vi "UserManage.vi"() -> ()   [LabVIEW 2011]
uses:
  Global/Globalclient.vi
panel:
  out "删除用户":string
  out "已登陆":string[][](table)
  in  "stop":bool
  out "未登陆":string[][](table)
  out "连接数":u8
  in  "Add Button":bool
  in  "Remove Button":bool
  out "射频":string[][](table)
  out "时钟":string[][](table)
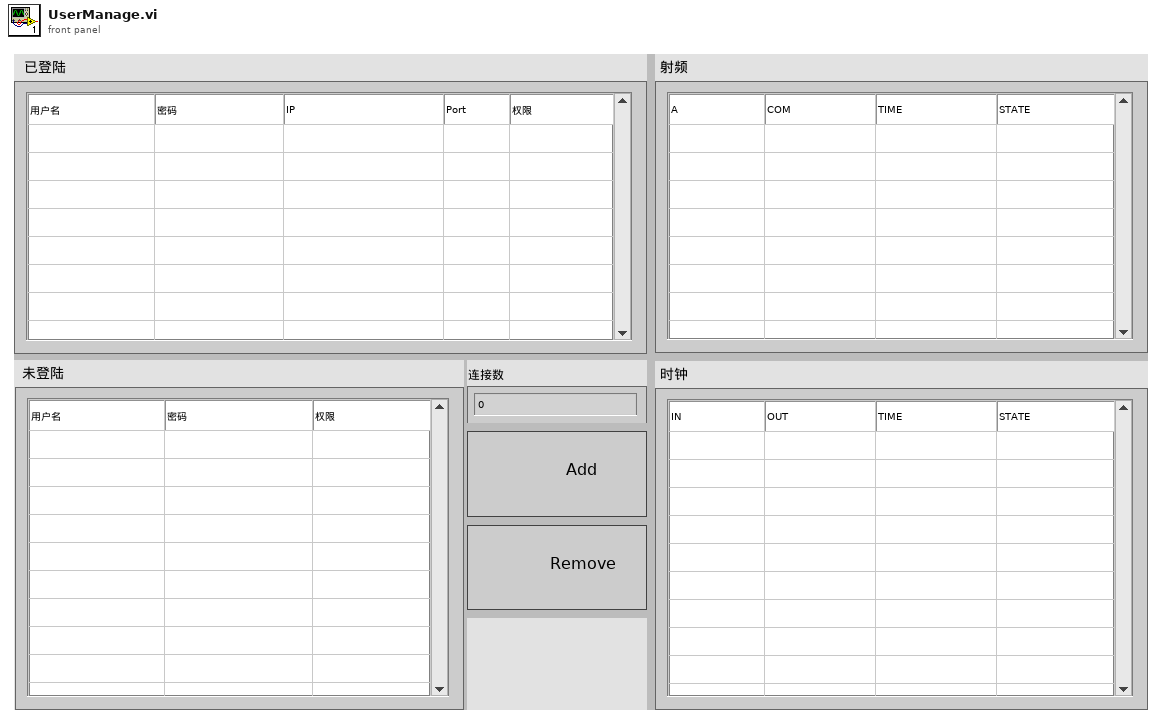
[diagram p1: front panel]
types:
  T1 = enum16{"Standard", "Buffered", "CRLF", "Immediate"}
  T2 = typedef "LVPoint32TypeDef.ctl" = cluster{"Horizontal":i32, "Vertical":i32}
  T3 = typedef "LVRowAndColumnTypeDef.ctl" = cluster{"Row":i32, "Column":i32}
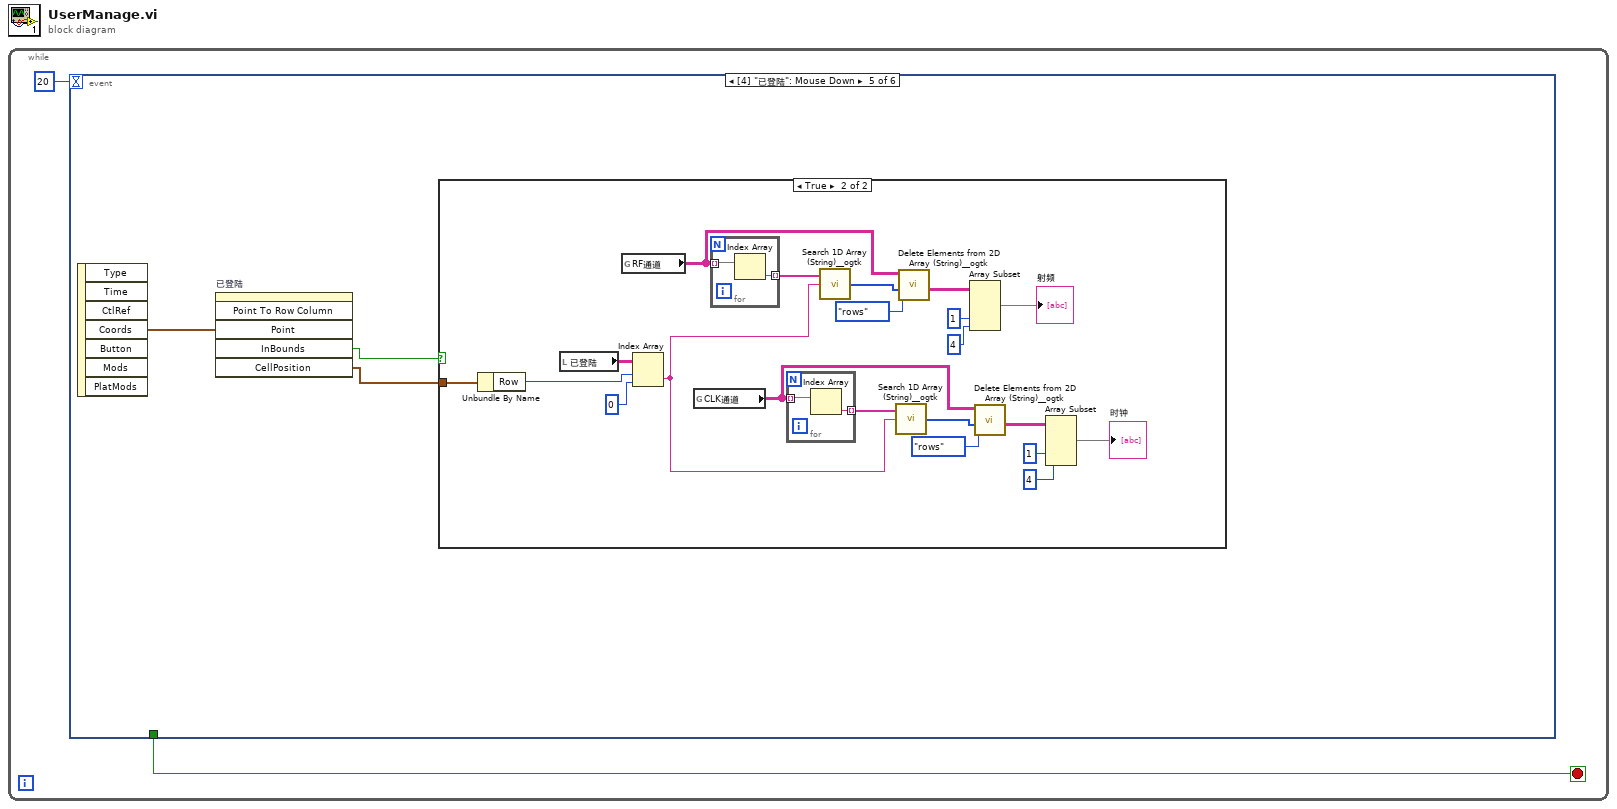
[diagram p0: block diagram]
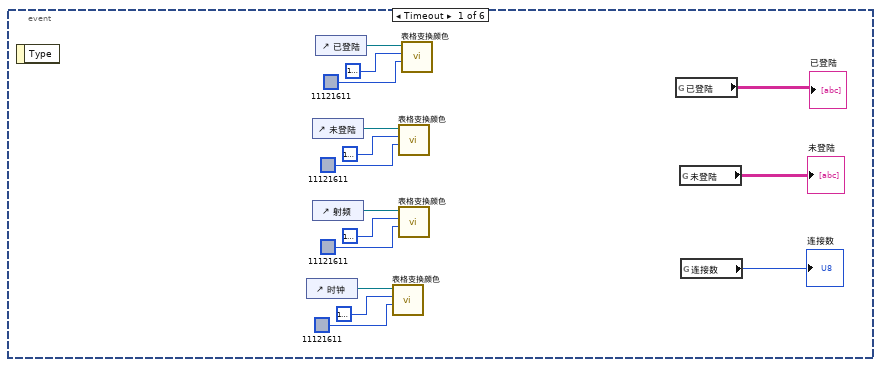
[diagram p2: hidden frame]
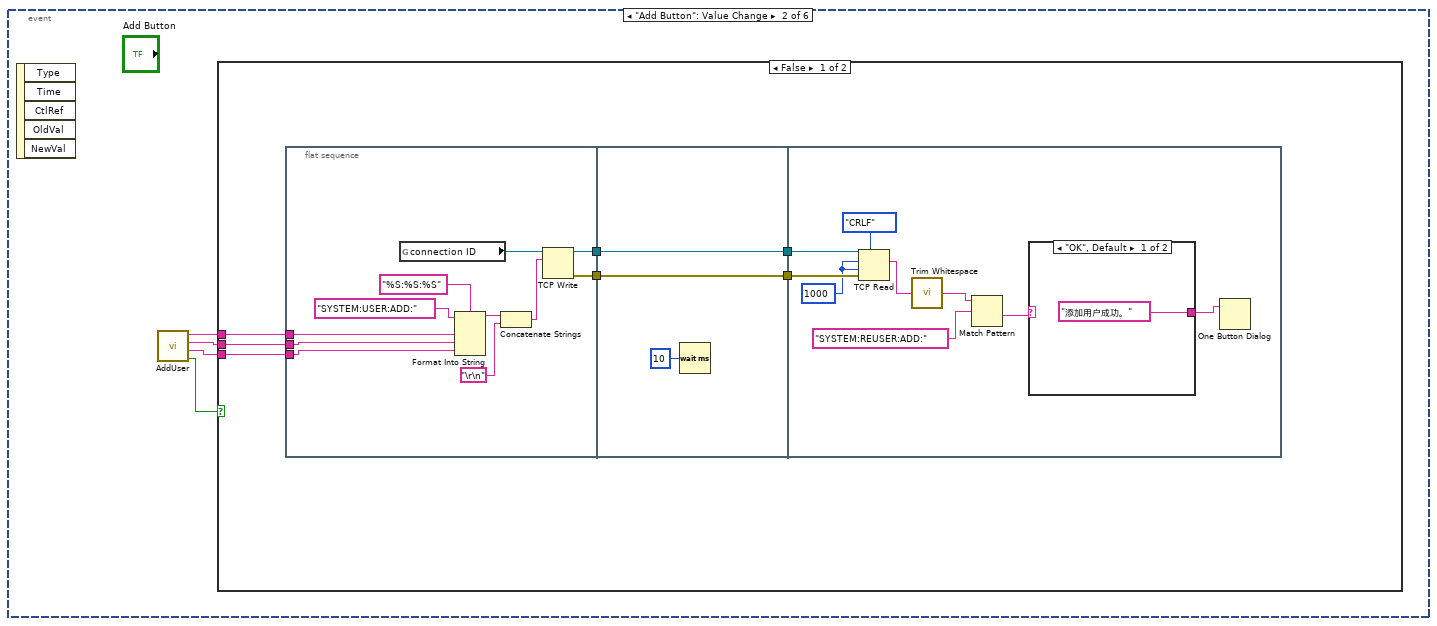
[diagram p3: hidden frame]
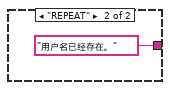
[diagram p4: hidden frame]
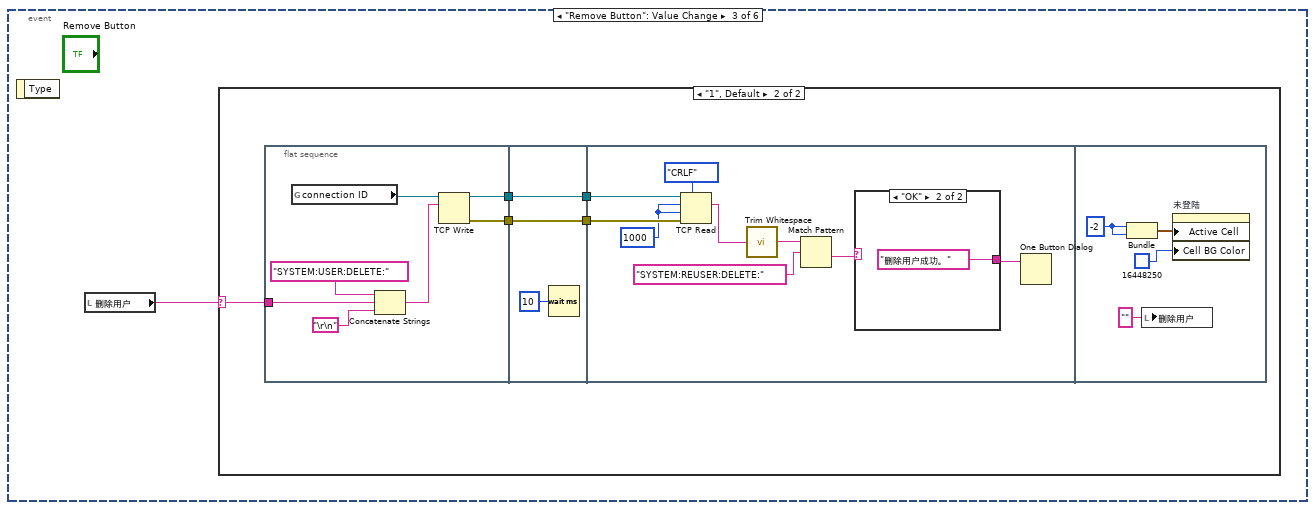
[diagram p6: hidden frame]
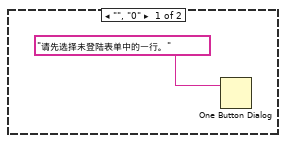
[diagram p7: hidden frame]
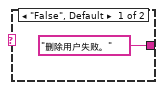
[diagram p8: hidden frame]
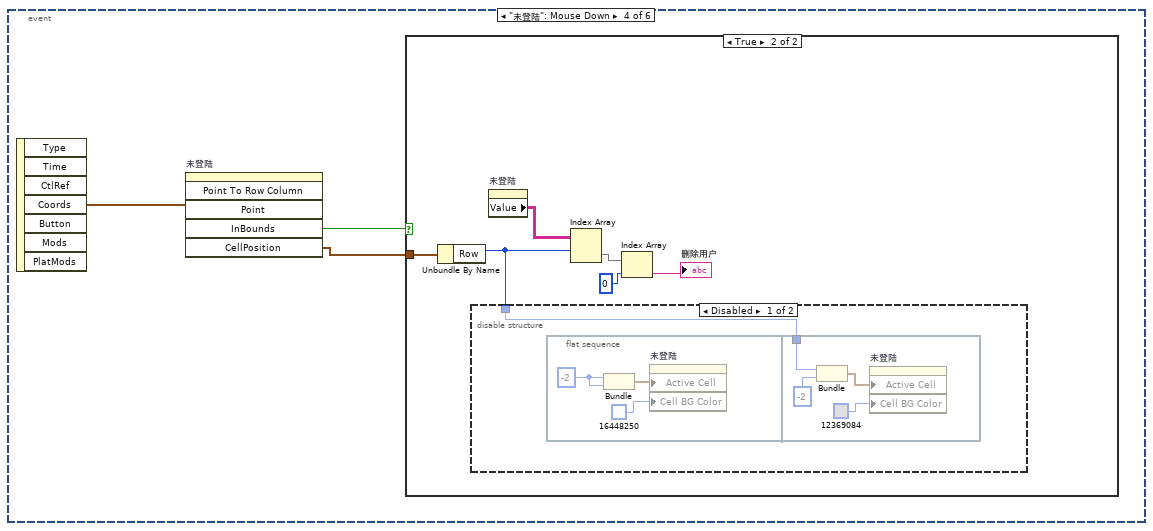
[diagram p9: hidden frame]
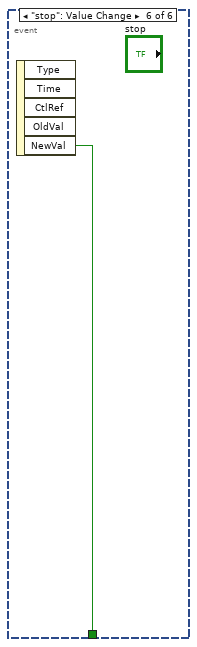
[diagram p13: hidden frame]
diagram:
  n1 = while {
    stop <- w2 stop-if-true
    n2 = event shown="[4] \"已登陆\": Mouse Down" {
      selector: _ -> [_ _ _ _ _ _]
      dyn-events: _ -> [_ _ _ _ _ _]
      timeout: 20 -> [_ _ _ _ _ _]
      tunnel: [_ _ _ _ _ w131] -> w2
      event Timeout {
        n3 = event-data() -> ()  [unwired: 1 in, 1 out]
        n4 = control-ref of="时钟"() -> (w7:refnum<vi>)
        n5 = control-ref of="未登陆"() -> (w13:refnum<vi>)
        n6 = control-ref of="射频"() -> (w12:refnum<vi>)
        n7 = control-ref of="已登陆"() -> (w3:refnum<vi>)
        n8 = call "表格变换颜色.vi"("奇数行背景颜色"=u32 11121611, "偶数行背景颜色"=u32 16777238, "MCListbox Refnum in"=w7) -> ()  [unwired: 7 in, 2 out]
        n9 = call "表格变换颜色.vi"("奇数行背景颜色"=u32 11121611, "偶数行背景颜色"=u32 16777238, "MCListbox Refnum in"=w13) -> ()  [unwired: 7 in, 2 out]
        n10 = call "表格变换颜色.vi"("奇数行背景颜色"=u32 11121611, "偶数行背景颜色"=u32 16777238, "MCListbox Refnum in"=w12) -> ()  [unwired: 7 in, 2 out]
        n11 = call "表格变换颜色.vi"("奇数行背景颜色"=u32 11121611, "偶数行背景颜色"=u32 16777238, "MCListbox Refnum in"=w3) -> ()  [unwired: 7 in, 2 out]
        n12 = global read "Globalclient.vi" "已登陆"() -> (→"已登陆":string[][])
        n13 = global read "Globalclient.vi" "未登陆"() -> (→"未登陆":string[][])
        n14 = global read "Globalclient.vi" "连接数"() -> (→"连接数":i32)
      }
      event "Add Button": Value Change {
        n15 = event-data() -> ()  [unwired: 1 in, 5 out]
        n16 = call "AddUser.vi"() -> ("drop?"=w21:bool, "Authority 2"=w18:string, "Password 2"=w19:string, "Username 2"=w20:string)  [unwired: 8 in]
        n17 = case shown="False" w21 {
          tunnel: w20 -> [w28 _]
          tunnel: w19 -> [w27 _]
          tunnel: w18 -> [w26 _]
          frame False {
            n18 = flat-sequence {
              tunnel: w28 -> [w36]
              tunnel: w27 -> [w35]
              tunnel: w26 -> [w34]
              tunnel: [w30] -> w24
              tunnel: [w29] -> w22
              tunnel: [w42] -> w25
              tunnel: w24 -> [w42]
              tunnel: [w41] -> w23
              tunnel: w22 -> [w41]
              tunnel: w25 -> [w51]
              tunnel: w23 -> [w50]
              frame #0 {
                n19 = global read "Globalclient.vi" "connection ID"() -> (w39:refnum<k5>)
                n20 = Format Into String(format string="%S:%S:%S", initial string="SYSTEM:USER:ADD:", w36, w35, w34) -> (resulting string=w33:string)  [unwired: 1 in, 1 out]
                n21 = Concatenate Strings(w33, "\r\n") -> (w31:string)
                n22 = TCP Write(connection ID=w39, data in=w31) -> (connection ID out=w30:refnum<k5>, error out=w29:errorcluster)  [unwired: 2 in, 1 out]
              }
              frame #1 {
                n23 = Wait (ms)(milliseconds to wait=u32 10) -> ()  [unwired: 1 out]
              }
              frame #2 {
                w49 = u32 1000 ("milliseconds to wait")
                n24 = TCP Read(connection ID=w51, bytes to read=w49, error in (no error)=w50, 7:T1."CRLF" ("mode (standard)"), 9:w49) -> (data out=w47:string)  [unwired: 2 out]
                n25 = call <vilib>:"Trim Whitespace.vi"("string"=w47) -> ("trimmed string"=w46:string)  [unwired: 1 in]
                n26 = Match Pattern(string=w46, regular expression="SYSTEM:REUSER:ADD:") -> (after substring=w44:string)  [unwired: 1 in, 3 out]
                n27 = case shown="\"OK\", Default" w44 {
                  tunnel: ["添加用户成功。" "用户名已经存在。"] -> w43
                  frame "OK", Default {
                  }
                  frame "REPEAT" {
                  }
                }
                n28 = One Button Dialog(message=w43) -> ()  [unwired: 1 in, 1 out]
              }
            }
          }
          frame True {
          }
        }
      }
      event "Remove Button": Value Change {
        n29 = event-data() -> ()  [unwired: 1 in, 1 out]
        n30 = local read "删除用户"() -> (w54:string)
        n31 = case shown="\"1\", Default" w54 {
          selector: w54 -> [_ w60]
          frame "", "0" {
            n32 = One Button Dialog(message="请先选择未登陆表单中的一行。") -> ()  [unwired: 1 in, 1 out]
          }
          frame "1", Default {
            n33 = flat-sequence {
              tunnel: w60 -> [w64]
              tunnel: [w62] -> w58
              tunnel: [w61] -> w56
              tunnel: [w70] -> w59
              tunnel: w58 -> [w70]
              tunnel: [w69] -> w57
              tunnel: w56 -> [w69]
              tunnel: w59 -> [w79]
              tunnel: w57 -> [w78]
              frame #0 {
                n34 = global read "Globalclient.vi" "connection ID"() -> (w67:refnum<k5>)
                n35 = Concatenate Strings("SYSTEM:USER:DELETE:", w64, "\r\n") -> (w63:string)
                n36 = TCP Write(connection ID=w67, data in=w63) -> (connection ID out=w62:refnum<k5>, error out=w61:errorcluster)  [unwired: 2 in, 1 out]
              }
              frame #1 {
                n37 = Wait (ms)(milliseconds to wait=u32 10) -> ()  [unwired: 1 out]
              }
              frame #2 {
                w76 = 1000
                n38 = TCP Read(connection ID=w79, bytes to read=w76, error in (no error)=w78, 7:T1."CRLF" ("mode (standard)"), 9:w76) -> (data out=w75:string)  [unwired: 2 out]
                n39 = call <vilib>:"Trim Whitespace.vi"("string"=w75) -> ("trimmed string"=w74:string)  [unwired: 1 in]
                n40 = Match Pattern(string=w74, regular expression="SYSTEM:REUSER:DELETE:") -> (after substring=w72:string)  [unwired: 1 in, 3 out]
                n41 = case shown="\"OK\"" w72 {
                  tunnel: ["删除用户失败。" "删除用户成功。"] -> w71
                  frame "False", Default {
                  }
                  frame "OK" {
                  }
                }
                n42 = One Button Dialog(message=w71) -> ()  [unwired: 1 in, 1 out]
              }
              frame #3 {
                w84 = -2 ("index")
                n43 = Bundle("index"=w84, "index"=w84) -> (w83:cluster{"index":i32, "index":i32})  [unwired: 1 in]
                n44 = local write "删除用户"("" ("删除用户")) -> ()
                n45 = property on="未登陆" class="Tbl (strict)"("Active Cell"=w83, "Cell BG Color"=u32 16448250) -> ()  [unwired: 2 in, 2 out]
              }
            }
          }
        }
      }
      event "未登陆": Mouse Down {
        n46 = event-data() -> ("Coords"=w88:T2)  [unwired: 1 in, 6 out]
        n47 = invoke on="未登陆" class="Tbl (strict)" method="Point To Row Column"("Point"=w88) -> ("InBounds"=w87:bool, "CellPosition"=w86:T3)  [unwired: 5 in, 4 out]
        n48 = case shown="True" w87 {
          tunnel: w86 -> [_ w94]
          frame False {
          }
          frame True {
            n49 = Unbundle By Name(w94) -> ("Row"=w89:i32)
            n50 = disable-structure shown="Disabled" {
              disable-tunnel: w89 -> [w95 _]
              frame Disabled {
                n51 = flat-sequence {
                  tunnel: w95 -> [w102]
                  frame #0 {
                    w98 = -2 ("index")
                    n52 = Bundle("index"=w98, "index"=w98) -> (w97:cluster{"index":i32, "index":i32})  [unwired: 1 in]
                    n53 = property on="未登陆" class="Tbl (strict)"("Active Cell"=w97, "Cell BG Color"=u32 16448250) -> ()  [unwired: 2 in, 2 out]
                  }
                  frame #1 {
                    n54 = Bundle("Row"=w102, "index"=-2) -> (w100:cluster{"Row":i32, "index":i32})  [unwired: 1 in]
                    n55 = property on="未登陆" class="Tbl (strict)"("Active Cell"=w100, "Cell BG Color"=u32 12369084) -> ()  [unwired: 2 in, 2 out]
                  }
                }
              }
              frame Enabled {
              }
            }
            n56 = property on="未登陆" class="Tbl (strict)"() -> ("Value"=w93:string[][])  [unwired: 2 in, 2 out]
            n57 = Index Array(array=w93, index (row)=w89) -> (element=w92:string[])  [unwired: 1 in]
            n58 = Index Array(array=w92, index=0) -> (element=→"删除用户":string)
          }
        }
      }
      event "已登陆": Mouse Down {
        n59 = event-data() -> ("Coords"=w105:T2)  [unwired: 1 in, 6 out]
        n60 = invoke on="已登陆" class="Tbl (strict)" method="Point To Row Column"("Point"=w105) -> ("InBounds"=w104:bool, "CellPosition"=w103:T3)  [unwired: 5 in, 4 out]
        n61 = case shown="True" w104 {
          tunnel: w103 -> [_ w126]
          frame False {
          }
          frame True {
            n62 = Unbundle By Name(w126) -> ("Row"=w124:i32)
            n63 = local read "已登陆"() -> (w125:string[][])
            n64 = global read "Globalclient.vi" "RF通道"() -> (w122:string[][])
            n65 = Index Array(array=w125, index (row)=w124, index (col)=0 ("disabled index (col)")) -> (element=w107:string)
            n66 = global read "Globalclient.vi" "CLK通道"() -> (w109:string[][])
            n67 = for {
              tunnel: w122 -> [w130] mode=indexing
              tunnel: [w129] -> w121 mode=indexing
              n68 = Index Array(array=w130) -> (element=w129:string)  [unwired: 1 in]
            }
            n69 = for {
              tunnel: w109 -> [w128] mode=indexing
              tunnel: [w127] -> w110 mode=indexing
              n70 = Index Array(array=w128) -> (element=w127:string)  [unwired: 1 in]
            }
            n71 = call <userlib>:"Search 1D Array (String)__ogtk.vi"("Array"=w121, "Element Data"=w107) -> ("Indices of Elements"=w120:i32[])  [unwired: 7 in]
            n72 = call <userlib>:"Search 1D Array (String)__ogtk.vi"("Array"=w110, "Element Data"=w107) -> ("Indices of Elements"=w111:i32[])  [unwired: 7 in]
            n73 = call <userlib>:"Delete Elements from 2D Array (String)__ogtk.vi"("delete (rows or columns)"=enum16{"rows", "columns"}."rows", "indices"=w120, "array"=w122) -> ("deleted elements"=w118:string[][])  [unwired: 7 in, 1 out]
            n74 = Array Subset(array=w118, index (col)=1 ("index"), length (col)=4 ("length")) -> (→"射频":string[][])  [unwired: 2 in]
            n75 = call <userlib>:"Delete Elements from 2D Array (String)__ogtk.vi"("delete (rows or columns)"=enum16{"rows", "columns"}."rows", "indices"=w111, "array"=w109) -> ("deleted elements"=w113:string[][])  [unwired: 7 in, 1 out]
            n76 = Array Subset(array=w113, index (col)=1 ("index"), length (col)=4 ("length")) -> (→"时钟":string[][])  [unwired: 2 in]
          }
        }
      }
      event "stop": Value Change {
        n77 = event-data() -> ("NewVal"=w131:bool)  [unwired: 1 in, 4 out]
      }
    }
  }
